vi "Reset Signal Configuration.vi"(8 "error in (no error)":errorcluster, 11 "signal configuration in":refnum<class "SV Signal.lvclass">) -> (0 "error out":errorcluster, 3 "signal configuration out":refnum<class "SV Signal.lvclass">)   [LabVIEW 2017, in "SV Signal.lvclass"]
uses:
  <vilib>/addons/_NISVFA/_Generation/Signal Generation/SV Signal/SV Signal.lvclass
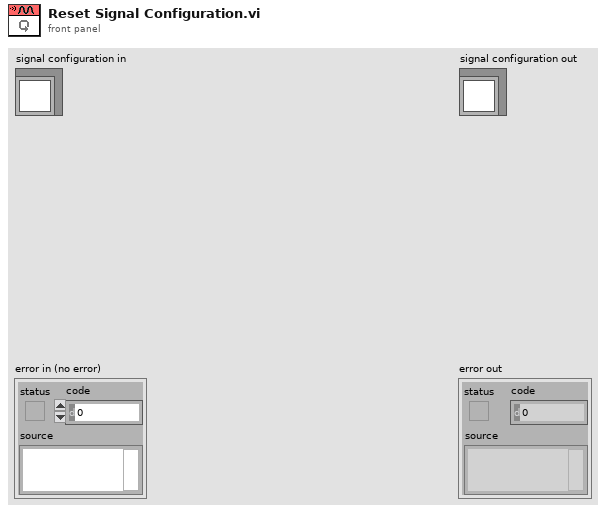
[diagram p1: front panel]
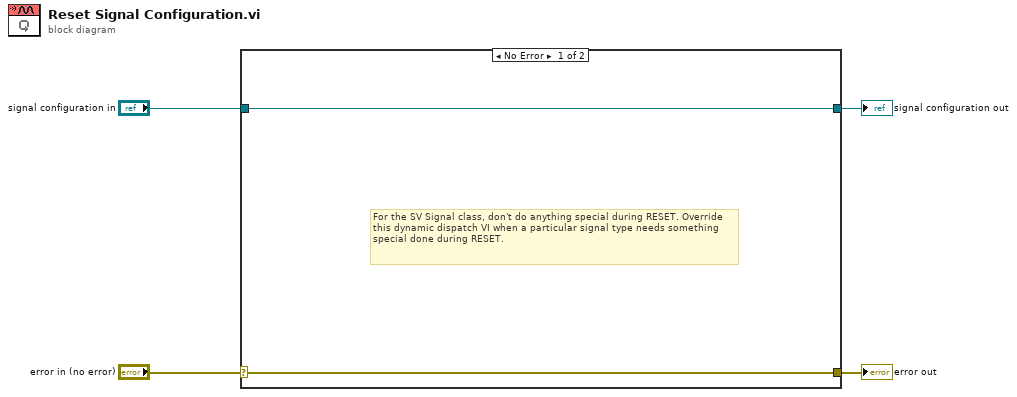
[diagram p0: block diagram]
diagram:
  n1 = case shown="No Error" "error in (no error)" {
    selector: "error in (no error)" -> [w5 w8]
    tunnel: [w5 w8] -> w3
    tunnel: [w6 w7] -> w1
    tunnel: "signal configuration in" -> [w6 w7]
    frame No Error {
      # "For the SV Signal class, don't do anything special during RESET. Override this dynamic dispatch VI when a particular signal type needs something special done during RESET."
    }
    frame Error {
    }
  }
  "error out" <- w3
  "signal configuration out" <- w1
